vi "subVI.vi"(10 "Numeric 2":dbl=6.0, 11 "Numeric":dbl=4.0) -> (3 "Numeric 3":dbl)   [LabVIEW 2015]
doc: "Mój pierwszy VI"
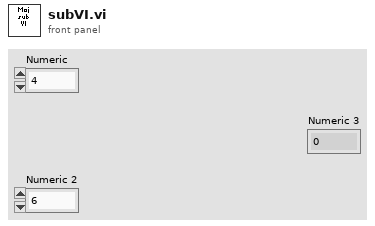
[diagram p1: front panel]
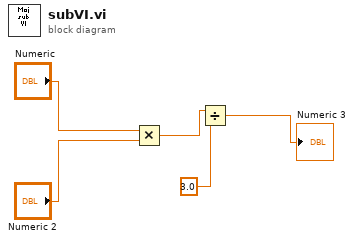
[diagram p0: block diagram]
diagram:
  n1 = Multiply(x="Numeric", y="Numeric 2") -> (x*y=w2:dbl)
  n2 = Divide(x=w2, y=3.0 ("x/y")) -> (x/y=→"Numeric 3":dbl)
